vi "BLAS1 Utility.vi"   [LabVIEW 2017, in "NI_AALBLAS.lvlib"]
uses:
  <vilib>/Analysis/NI_AALBLAS.lvlib
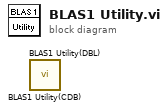
[diagram p0: block diagram]
diagram:
  n1 = call <vilib>:"BLAS1 Utility(CDB).vi"() -> ()  [unwired: 19 in, 1 out]
  n2 = call <vilib>:"BLAS1 Utility(DBL).vi"() -> ()  [unwired: 19 in, 1 out]
